vi "bottle filler sim.vi"() -> ()   [LabVIEW 2009]
panel:
  out "motor running?(no:F)":bool
  out "status":T1(ring)
  out "bottles filled":dbl
  in  "PROXIMITY bottle in position (V)":dbl(slide)
  in  "FILL load cell (V)":dbl(slide)
  in  "stop":bool
  out "6 bottles in place?(no:F)":bool
  in  "bottle Cluster":T2
  # "here is a simulation of a bottle filler:\n\n1) RUN vi\n2) Place bottles into system by pressing all buttons \n3) motor will run, until proximity voltage is reached\n4) water valve opens until load cell voltage is reached, increment bottles filled\n5) goto step 3, until 6 bottles filled, then shutdown system"
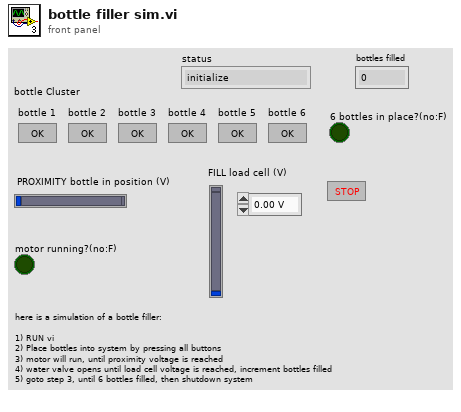
[diagram p1: front panel]
types:
  T1 = enum16{"initialize", "wait", "fill", "bottle in position", "shutdown"}
  T2 = cluster{"bottle 1":bool, "bottle 2":bool, "bottle 3":bool, "bottle 4":bool, "bottle 5":bool, "bottle 6":bool}
  T3 = cluster{"[0]":bool, "[1]":bool, "[2]":bool, "[3]":bool, "[4]":bool, "[5]":bool}
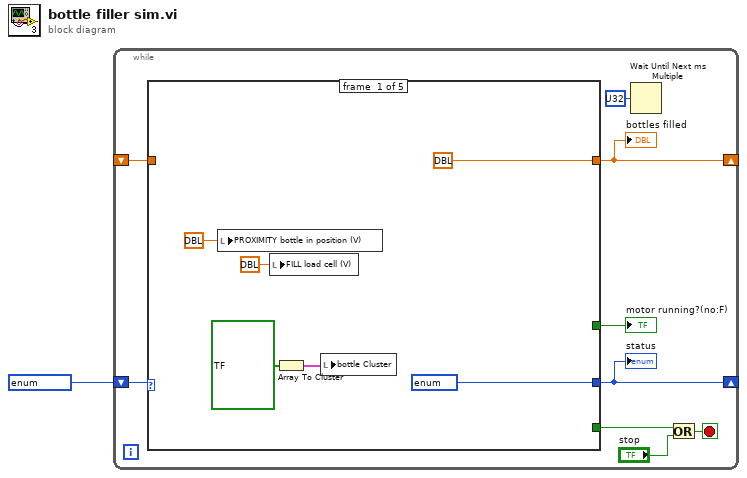
[diagram p0: block diagram]
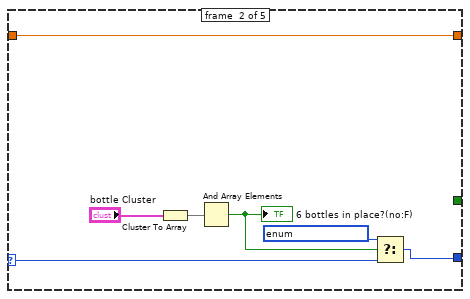
[diagram p2: hidden frame]
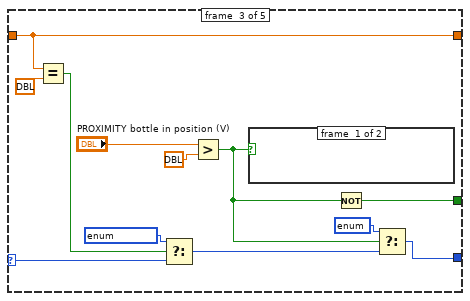
[diagram p3: hidden frame]
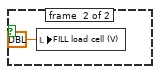
[diagram p4: hidden frame]
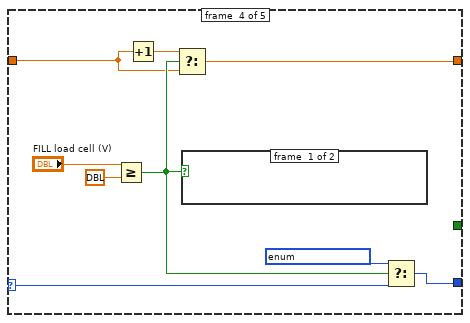
[diagram p5: hidden frame]
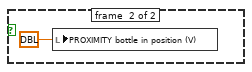
[diagram p6: hidden frame]
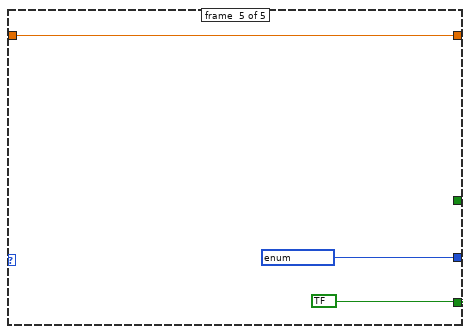
[diagram p7: hidden frame]
diagram:
  n1 = while {
    shift-right: [w8] -> _
    shift-left: _ -> [w7]
    shift-right: [w5] -> _
    shift-left: T1 ? -> [w6]
    stop <- w4 stop-if-true
    n2 = case shown="\"wait\"" w6 {
      selector: w6 -> [_ w22 w28 w37 _]
      tunnel: [dbl ? w23 w30 w40 w49] -> w8
      tunnel: w7 -> [_ w23 w30 w38 w49]
      tunnel: [T1 ? ("t") w21 w35 w45 T1 ? ("t")] -> w5
      tunnel: [_ _ _ _ bool ?] -> w3
      tunnel: [_ _ w24 _ _] -> w2
      frame #0 {
        n3 = local write "PROXIMITY bottle in position (V)"(dbl ? ("bottle in position (V)")) -> ()
        n4 = local write "FILL load cell (V)"(dbl ? ("load cell (V)")) -> ()
        n5 = Array To Cluster(array=bool[] ?) -> (cluster=w13:T3)
        n6 = local write "bottle Cluster"(w13) -> ()
      }
      frame #1 {
        n7 = Cluster To Array(cluster="bottle Cluster") -> (array=w19:bool[])
        n8 = And Array Elements(Boolean array=w19) -> (logical AND=w18:bool)
        "6 bottles in place?(no:F)" <- w18
        n9 = Select(t=T1 ?, s=w18, f=w22) -> (s? t:f=w21:T1)
      }
      frame #2 {
        n10 = Equal?(x=w30, y=dbl ?) -> (x = y?=w27:bool)
        n11 = Select(t=T1 ?, s=w27, f=w28) -> (s? t:f=w26:T1)
        n12 = Greater?(x="PROXIMITY bottle in position (V)", y=dbl ?) -> (0:w25:bool)
        n13 = case shown="True" w25 {
          frame #0 {
          }
          frame #1 {
            n14 = local write "FILL load cell (V)"(dbl ? ("load cell (V)")) -> ()
          }
        }
        n15 = Not(x=w25) -> (.not. x?=w24:bool)
        n16 = Select(t=T1 ?, s=w25, f=w26) -> (s? t:f=w35:T1)
      }
      frame #3 {
        n17 = Greater Or Equal?(x="FILL load cell (V)", y=dbl ?) -> (x >= y?=w39:bool)
        n18 = Increment(x=w38) -> (x+1=w41:dbl)
        n19 = Select(t=w41, s=w39, f=w38) -> (s? t:f=w40:dbl)
        n20 = case shown="True" w39 {
          frame #0 {
          }
          frame #1 {
            n21 = local write "PROXIMITY bottle in position (V)"(dbl ? ("bottle in position (V)")) -> ()
          }
        }
        n22 = Select(t=T1 ?, s=w39, f=w37) -> (s? t:f=w45:T1)
      }
      frame #4 {
      }
    }
    "bottles filled" <- w8
    "status" <- w5
    "motor running?(no:F)" <- w2
    n23 = Wait Until Next ms Multiple(millisecond multiple=u32 ?) -> ()  [unwired: 1 out]
    n24 = Or(x=w3, y="stop") -> (x .or. y?=w4:bool)
  }
